vi "s7ice.vi"() -> ()   [LabVIEW 2024]
panel:
  out "2D Picture":picture
  in  "Slide":dbl(slide) scale=0.0..10.0
  in  "stop":bool
  in  "ActiveX Container":refnum<k7>(container)
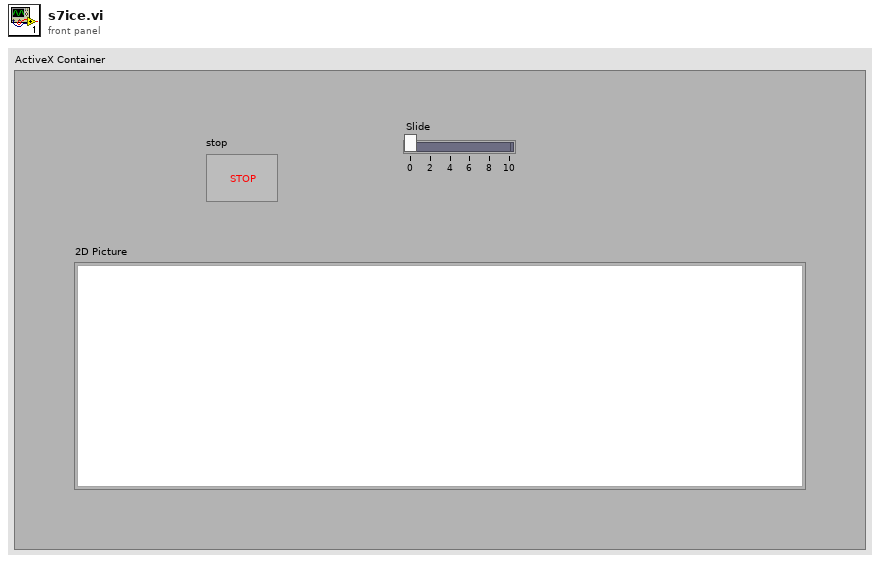
[diagram p1: front panel]
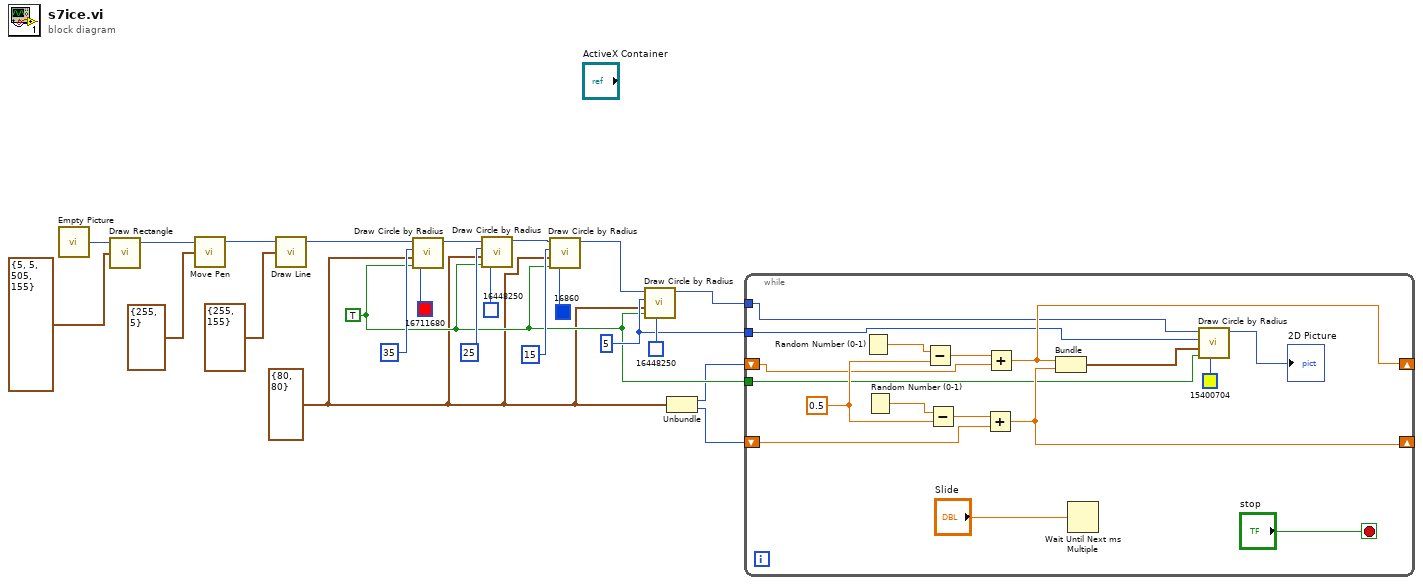
[diagram p0: block diagram]
diagram:
  w8 = cluster{i32, i32} {80, 80}
  w11 = TRUE
  w12 = 5
  n1 = call "Empty Picture"() -> ("empty picture"=w1:picture)
  n2 = call <vilib>:"Draw Rectangle.vi"("picture"=w1, "rect"=cluster{i32, i32, i32, i32} {5, 5, 505, 155}) -> ("new picture"=w3:picture)  [unwired: 7 in]
  n3 = call <vilib>:"Move Pen.vi"("new position"=cluster{i32, i32} {255, 5}, "picture"=w3) -> ("new picture"=w5:picture)  [unwired: 3 in]
  n4 = call <vilib>:"Draw Line.vi"("picture"=w5, "end point"=cluster{i32, i32} {255, 155}) -> ("new picture"=w7:picture)  [unwired: 7 in]
  n5 = call <vilib>:"Draw Circle by Radius.vi"("color(black)"=u32 16711680, "fill?(F)"=w11, "pixel center"=w8, "radius"=35, "picture"=w7) -> ("new picture"=w15:picture)  [unwired: 6 in]
  n6 = call <vilib>:"Draw Circle by Radius.vi"("color(black)"=u32 16448250, "fill?(F)"=w11, "pixel center"=w8, "radius"=25, "picture"=w15) -> ("new picture"=w14:picture)  [unwired: 6 in]
  n7 = call <vilib>:"Draw Circle by Radius.vi"("color(black)"=u32 16860, "fill?(F)"=w11, "pixel center"=w8, "radius"=15, "picture"=w14) -> ("new picture"=w13:picture)  [unwired: 6 in]
  n8 = call <vilib>:"Draw Circle by Radius.vi"("color(black)"=u32 16448250, "fill?(F)"=w11, "pixel center"=w8, "radius"=w12, "picture"=w13) -> ("new picture"=w16:picture)  [unwired: 6 in]
  n9 = Unbundle(w8) -> (w10:i32, w9:i32)
  n10 = while {
    shift-right: [w30] -> _
    shift-left: w10 -> [w25]
    shift-right: [w29] -> _
    shift-left: w9 -> [w24]
    tunnel: w16 -> [w28]
    tunnel: w12 -> [w27]
    tunnel: w11 -> [w26]
    stop <- "stop" stop-if-true
    w32 = 0.5
    n11 = Random Number (0-1)() -> (number: 0 to 1=w36:dbl)
    n12 = Random Number (0-1)() -> (number: 0 to 1=w34:dbl)
    n13 = Subtract(x=w36, y=w32) -> (x-y=w35:dbl)
    n14 = Subtract(x=w34, y=w32) -> (x-y=w33:dbl)
    n15 = Add(x=w33, y=w24) -> (x+y=w29:dbl)
    n16 = Add(x=w35, y=w25) -> (x+y=w30:dbl)
    n17 = Bundle(w30, w29) -> (w31:cluster{dbl, dbl})  [unwired: 1 in]
    n18 = Wait Until Next ms Multiple(millisecond multiple="Slide") -> ()  [unwired: 1 out]
    n19 = call <vilib>:"Draw Circle by Radius.vi"("color(black)"=u32 15400704, "fill?(F)"=w26, "pixel center"=w31, "radius"=w27, "picture"=w28) -> ("new picture"=→"2D Picture":picture)  [unwired: 6 in]
  }
